vi "interpolation.vi"(9 "position":dbl, 10 "Up":dbl, 11 "Down":dbl) -> (3 "Output":dbl)   [LabVIEW 2013]
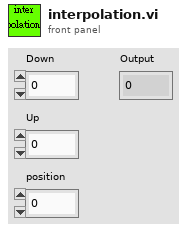
[diagram p1: front panel]
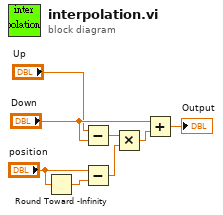
[diagram p0: block diagram]
diagram:
  n1 = Round Toward -Infinity(1:"position") -> (0:w5:dbl)
  n2 = Subtract(x="Up", y="Down") -> (x-y=w1:dbl)
  n3 = Subtract(x="position", y=w5) -> (x-y=w2:dbl)
  n4 = Multiply(x=w1, y=w2) -> (x*y=w3:dbl)
  n5 = Add(x="Down", y=w3) -> (x+y=→"Output":dbl)
